vi "Enqueue in Front.vi"(8 "error in (no error)":errorcluster, 9 "Message Priority":T1=enum."Normal", 10 "Message":refnum<class "Message.lvclass">, 11 "Sequencer Core in":refnum<class "Sequencer Core.lvclass">) -> (0 "error out":errorcluster, 3 "Sequencer Core out":refnum<class "Sequencer Core.lvclass">)   [LabVIEW 2020, in "Sequencer.lvlib" / "Sequencer Core.lvclass"]
doc: "Enqueue a message element in front on the Sequencer Core."
uses:
  Sequencer Core.lvclass
  PPL/HDH.Actor Framework.Core.Actor.lvlibp/1abvi3w/vi.lib/ActorFramework/Message Enqueuer/Message Priority.ctl
  PPL/HDH.Actor Framework.Core.Actor.lvlibp/1abvi3w/vi.lib/ActorFramework/Message/Message.lvclass
  Sequencer Core.lvclass/Sequencer Core.ctl
  Message Priority Queue/Message Priority Queue.lvclass
  PPL/HDH.Actor Framework.Core.Actor.lvlibp/1abvi3w/vi.lib/ActorFramework/Message Enqueuer/Message Enqueuer.lvclass
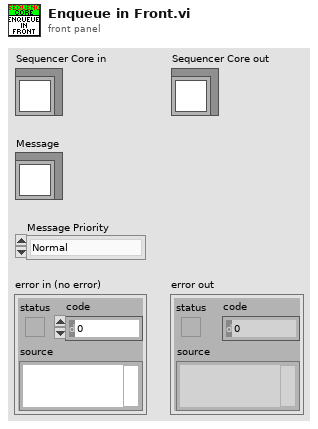
[diagram p1: front panel]
types:
  T1 = typedef "HDH.Actor Framework.Core.Actor.lvlibp/Message Enqueuer.lvclass/Message Priority.ctl" = enum16{"Low", "Normal", "High"}
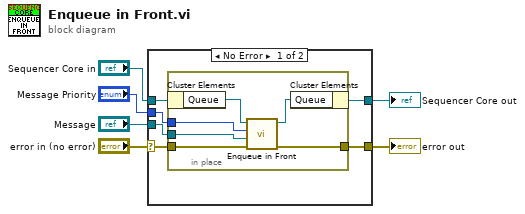
[diagram p0: block diagram]
diagram:
  n1 = case shown="No Error" "error in (no error)" {
    selector: "error in (no error)" -> [w11 w20]
    tunnel: [w10 w20] -> w5
    tunnel: [w7 w19] -> w3
    tunnel: "Sequencer Core in" -> [w12 w19]
    tunnel: "Message" -> [w9 _]
    tunnel: "Message Priority" -> [w8 _]
    frame No Error {
      n2 = in-place {
        in-place-border: w11 -> [w17]
        in-place-border: [w16] -> w10
        in-place-border: w9 -> [w14]
        in-place-border: w8 -> [w15]
        n3 = in-place-cluster #1(w12) -> ("Queue"=w13:refnum<class "Message Priority Queue.lvclass">)
        n4 = call "Enqueue in Front.vi"("error in (no error)"=w17, "Message"=w14, "priority"=w15, "Priority Queue in"=w13) -> ("error out"=w16:errorcluster, "Priority Queue out"=w18:refnum<class "Message Priority Queue.lvclass">)  [unwired: 6 in]
        n5 = in-place-cluster #1("Queue"=w18) -> (w7:refnum<class "Sequencer Core.lvclass">)
      }
    }
    frame Error {
    }
  }
  "error out" <- w5
  "Sequencer Core out" <- w3
